vi "Initialize XNET Tree.vi"(4 "Info?":refnum<vi>, 6 "Node Ptr":u64 format="%.0x", 8 "error in":errorcluster, 9 "XNET Cluster":refnum<k21>, 10 "XNET Database":refnum<k21>, 11 "Tree":refnum<vi>) -> (0 "error out":errorcluster, 1 "Parent":string, 2 "XNET Cluster Out":refnum<k21>, 3 "Tree Out":refnum<vi>)   [LabVIEW 2023, in "Protection and Counter Addon System Explorer.lvlib"]
uses:
  Protection and Counter Addon System Explorer.lvlib
  Types/CAN Filter Type.ctl
  Addon Shared/SubVIs/GUID Lookup.vi
  <resource>/objmgr/xnet.rc
  <vilib>/NI VeriStand/Custom Device API/Custom Device API.lvlib
  Addon Shared/Protection and Counter Addon Shared.lvlib
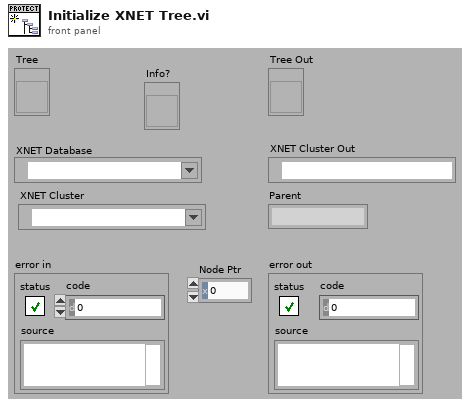
[diagram p1: front panel]
types:
  T1 = typedef "Protection and Counter Addon System Explorer.lvlib/CAN Filter Type.ctl" = enum16{"Cyclic Data", "Event Data", "Cyclic/Event", "All"}
  T2 = typedef "Custom Device API.lvlib/Custom Device Item Info.ctl" = cluster{"Name":string, "Is Channel":bool, "GUID":string, "Is Waveform":bool}
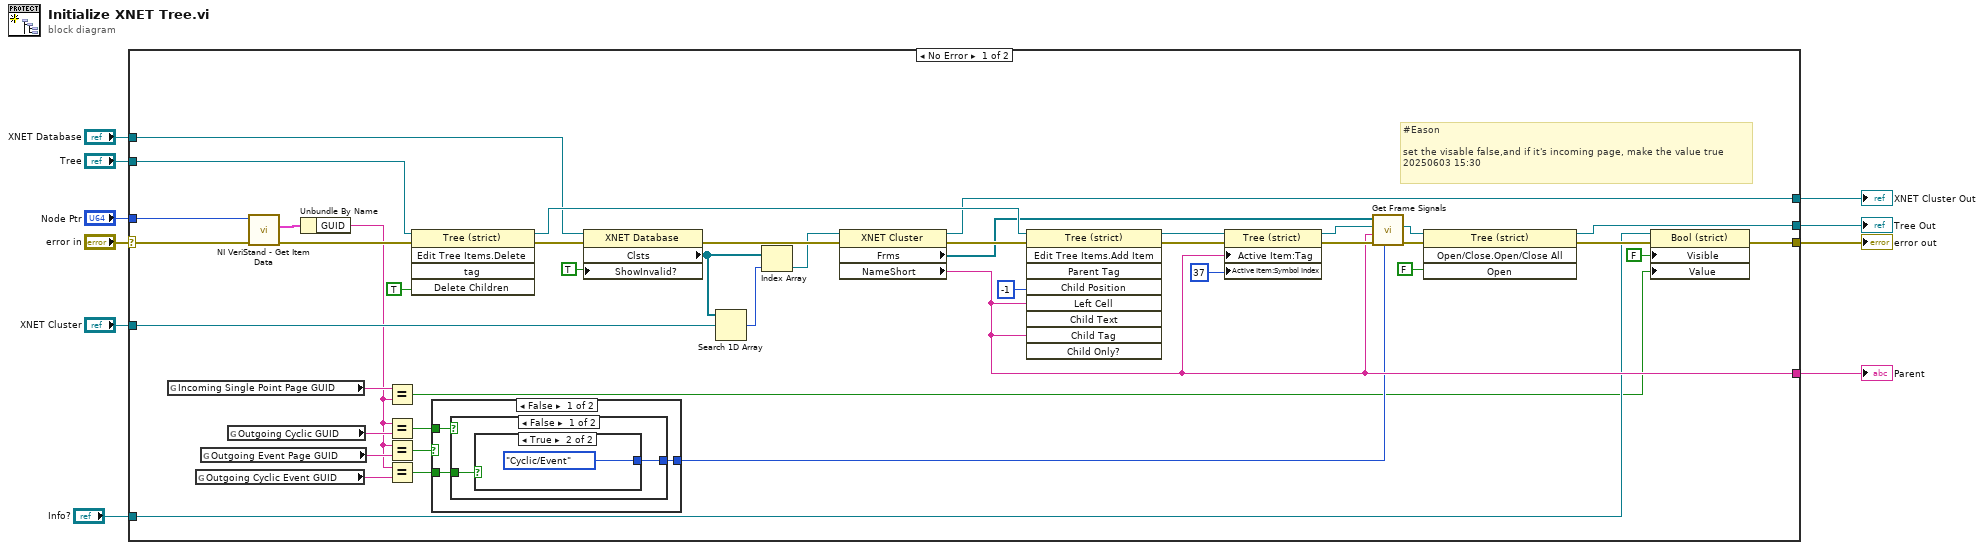
[diagram p0: block diagram]
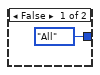
[diagram p2: hidden frame]
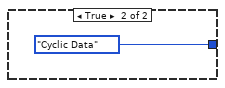
[diagram p3: hidden frame]
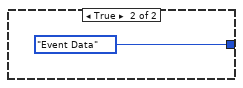
[diagram p4: hidden frame]
diagram:
  n1 = case shown="No Error" "error in" {
    selector: "error in" -> [w28 w65]
    tunnel: "Tree" -> [w52 w64]
    tunnel: [w20 w65] -> w9
    tunnel: "XNET Database" -> [w37 _]
    tunnel: [w40 w64] -> w6
    tunnel: [w42 w63] -> w5
    tunnel: "XNET Cluster" -> [w33 w63]
    tunnel: [w29 _] -> w3
    tunnel: "Node Ptr" -> [w26 _]
    tunnel: "Info?" -> [w19 _]
    frame No Error {
      # "#Eason\n\nset the visable false,and if it's incoming page, make the value true \n20250603 15:30"
      n2 = global read "GUID Lookup.vi" "Incoming Single Point Page GUID"() -> (w18:string)
      n3 = global read "GUID Lookup.vi" "Outgoing Cyclic Event GUID"() -> (w15:string)
      n4 = global read "GUID Lookup.vi" "Outgoing Event Page GUID"() -> (w16:string)
      n5 = global read "GUID Lookup.vi" "Outgoing Cyclic GUID"() -> (w17:string)
      n6 = call <vilib>:"NI VeriStand - Get Item Data.vi"("error in (no error)"=w28, "Item Ref in"=w26) -> ("error out"=w27:errorcluster, "Item Info"=w25:T2)  [unwired: 6 in, 2 out]
      n7 = Unbundle By Name(w25) -> ("GUID"=w14:string)
      n8 = Equal?(x=w18, y=w14) -> (x = y?=w12:bool)
      n9 = Equal?(x=w14, y=w17) -> (x = y?=w23:bool)
      n10 = Equal?(x=w14, y=w16) -> (x = y?=w24:bool)
      n11 = Equal?(x=w14, y=w15) -> (x = y?=w13:bool)
      n12 = invoke on="Invoke Node" class="Tree (strict)" method="Edit Tree Items.Delete"(reference=w52, error in=w27, "Delete Children"=TRUE ("Delete Children?")) -> (reference out=w53:refnum<vi>, error out=w35:errorcluster)  [unwired: 2 in, 3 out]
      n13 = case shown="False" w24 {
        tunnel: w23 -> [w56 _]
        tunnel: [w55 CAN_Filter_Type."Event Data" ("CAN:Frame Type")] -> w22
        tunnel: w13 -> [w54 _]
        frame False {
          n14 = case shown="False" w56 {
            tunnel: [w58 CAN_Filter_Type."Cyclic Data" ("CAN:Frame Type")] -> w55
            tunnel: w54 -> [w57 _]
            frame False {
              n15 = case shown="True" w57 {
                tunnel: [CAN_Filter_Type."All" ("CAN:Frame Type") CAN_Filter_Type."Cyclic/Event" ("CAN:Frame Type")] -> w58
                frame False {
                }
                frame True {
                }
              }
            }
            frame True {
            }
          }
        }
        frame True {
        }
      }
      n16 = property class="XNET Database"(reference=w37, error in=w35, "ShowInvalid?"=TRUE ("Show Invalid From Open?")) -> (error out=w34:errorcluster, "Clsts"=w31:refnum<k21>[])  [unwired: 1 out]
      n17 = Search 1D Array(1D array=w31, element=w33) -> (index of element=w32:i32)  [unwired: 1 in]
      n18 = Index Array(array=w31, index=w32) -> (element=w30:refnum<k21>)
      n19 = property class="XNET Cluster"(reference=w30, error in=w34) -> (reference out=w42:refnum<k21>, error out=w44:errorcluster, "Frms"=w43:refnum<k21>[], "NameShort"=w29:string)
      n20 = invoke on="Invoke Node" class="Tree (strict)" method="Edit Tree Items.Add Item"(reference=w53, error in=w44, "Child Position"=-1, "Left Cell"=w29, "Child Tag"=w29) -> (reference out=w47:refnum<vi>, error out=w46:errorcluster)  [unwired: 4 in, 7 out]
      n21 = property class="Tree (strict)"(reference=w47, error in=w46, "Active Item:Tag"=w29, "Active Item:Symbol Index"=37) -> (reference out=w48:refnum<vi>, error out=w49:errorcluster)
      n22 = call "Get Frame Signals.vi"("CAN:Frame Type"=w22, "error in"=w49, "Parent Tag"=w29, "Tree Reference"=w48, "Frms"=w43) -> ("error out"=w39:errorcluster, "Tree Reference Out"=w38:refnum<vi>)  [unwired: 5 in]
      n23 = invoke on="Invoke Node" class="Tree (strict)" method="Open/Close.Open/Close All"(reference=w38, error in=w39, "Open"=FALSE ("Open?")) -> (reference out=w40:refnum<vi>, error out=w21:errorcluster)  [unwired: 1 in, 2 out]
      n24 = property class="Bool (strict)"(reference=w19, error in=w21, "Visible"=FALSE, "Value"=w12) -> (error out=w20:errorcluster)  [unwired: 1 out]
    }
    frame Error {
    }
  }
  "error out" <- w9
  "Tree Out" <- w6
  "XNET Cluster Out" <- w5
  "Parent" <- w3
